vi "S2DS_Get system file (SubVI).vi"(8 "error in (no error)":errorcluster) -> (0 "error out":errorcluster, 3 "Refnum out":T1)   [LabVIEW 2025]
uses:
  <vilib>/Utility/config.llb/Config Data RefNum.ctl
  <vilib>/Utility/sysdir.llb/System Directory Type.ctl
  <vilib>/Utility/config.llb/NI_LVConfig.lvlib
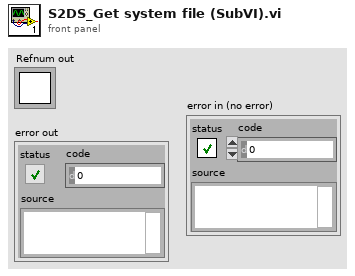
[diagram p1: front panel]
types:
  T1 = typedef "NI_LVConfig.lvlib/Config Data RefNum.ctl" = refnum<k1>
  T2 = typedef "System Directory Type.ctl" = i32
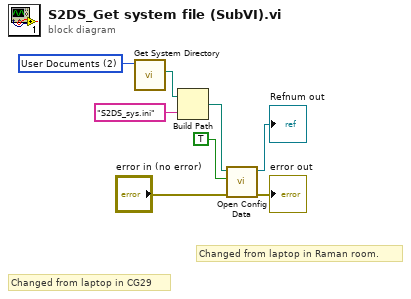
[diagram p0: block diagram]
diagram:
  w3 = T2 2 items=["User Home"=0, "User Desktop"=1, "User Documents"=2, "User Application Data"=3, "User Preferences"=4, "User Temporary"=5, "Public Documents"=6, "Public Application Data"=7, "Public Preferences"=8, "Public Cache"=13, "System Core Libraries"=9, "System Installed Libraries"=10, "Application Files"=11, "Boot Volume Root"=12] ("system directory type")
  # "Changed from laptop in CG29"
  # "Changed from laptop in Raman room."
  n1 = call <vilib>:"Get System Directory.vi"("system directory type"=w3) -> ("system directory"=w4:path)  [unwired: 10 in]
  n2 = Build Path(base path=w4, name or relative path="S2DS_sys.ini") -> (appended path=w6:path)
  n3 = call <vilib>:"Open Config Data.vi"("error in (no error)"="error in (no error)", "create file if necessary (T)"=TRUE, "configuration file path"=w6) -> ("error out"=→"error out":errorcluster, "refnum"=→"Refnum out":T1)  [unwired: 6 in, 1 out]
